vi "DPO_7K_Enable_Channel.vi"(8 "Error In":errorcluster, 9 "Activate?":bool, 10 "Channel":u16(ring) items=["Channel 1", "Channel 2", "Channel 3", "Channel 4", "Math 1", "Math 2", "Math 3", "Math 4", "Reference 1", "Reference 2", "Reference 3", "Reference 4"], 11 "VISA resource name in":refnum<visa-resource-name>) -> (0 "Error Out":errorcluster, 2 "State_Channel":bool, 3 "VISA resource name out":refnum<visa-resource-name>)   [LabVIEW 2020]
panel:
  out "concatenated string":string
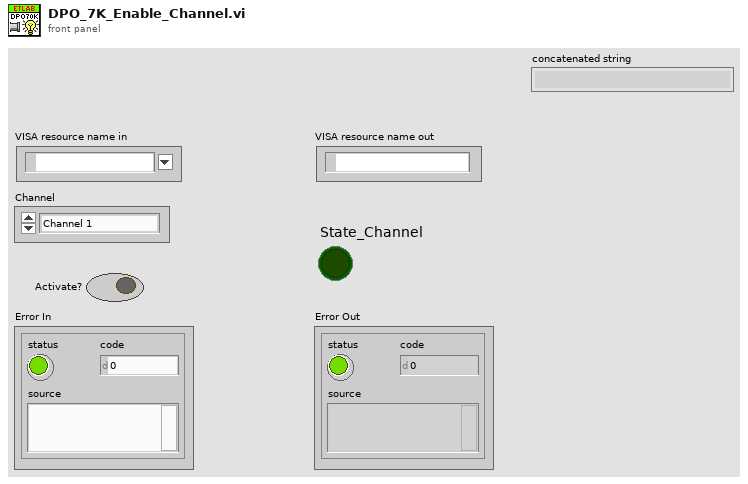
[diagram p1: front panel]
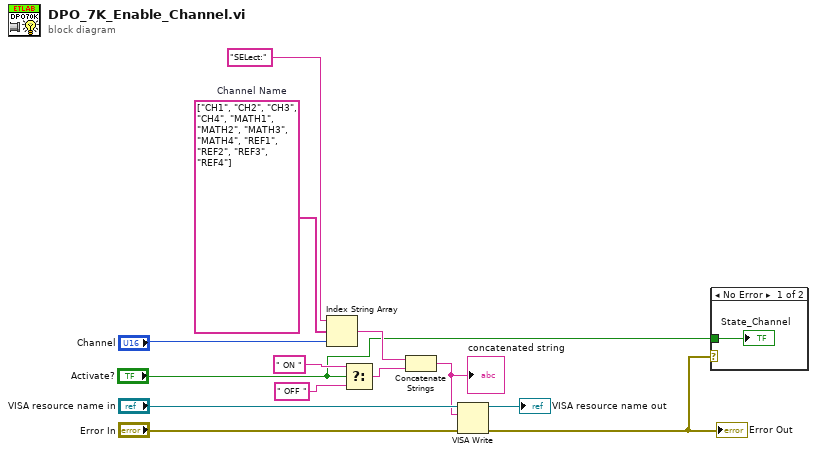
[diagram p0: block diagram]
diagram:
  w11 = string[] ["CH1", "CH2", "CH3", "CH4", "MATH1", "MATH2", "MATH3", "MATH4", "REF1", "REF2", "REF3", "REF4"]  # Channel Name
  n1 = Index String Array(1:"Channel", 2:w11, 3:"SELect:") -> (0:w7:string)
  n2 = Select(t=" ON ", s="Activate?", f=" OFF ") -> (s? t:f=w4:string)
  n3 = Concatenate Strings(w7, w4) -> (w6:string)
  "concatenated string" <- w6
  n4 = VISA Write(VISA resource name="VISA resource name in", write buffer=w6, error in (no error)="Error In") -> (VISA resource name out=→"VISA resource name out":refnum<visa-resource-name>, error out=w2:errorcluster)  [unwired: 1 out]
  "Error Out" <- w2
  n5 = case shown="No Error" w2 {
    tunnel: "Activate?" -> [w14 _]
    frame No Error {
      "State_Channel" <- w14
    }
    frame Error {
    }
  }
